vi "Compond_arithmetic.vi"() -> ()   [LabVIEW 2019]
panel:
  out "Result":bool
  in  "Boolean 4":bool
  in  "Boolean 3":bool
  in  "Boolean 2":bool
  in  "Boolean":bool
  # "Only for Boolean Operators"
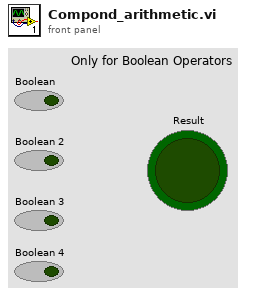
[diagram p1: front panel]
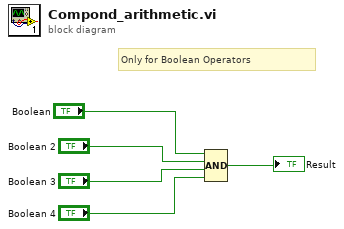
[diagram p0: block diagram]
diagram:
  # "Only for Boolean Operators"
  n1 = Compound Arithmetic op=AND("Boolean", "Boolean 2", "Boolean 3", "Boolean 4") -> (→"Result":bool)
